vi "Average temperature.vi"() -> ()   [LabVIEW 2019]
panel:
  out "Waveform Chart":cluster{dbl, "Temperature":dbl}(graph)
  in  "Вкл":bool
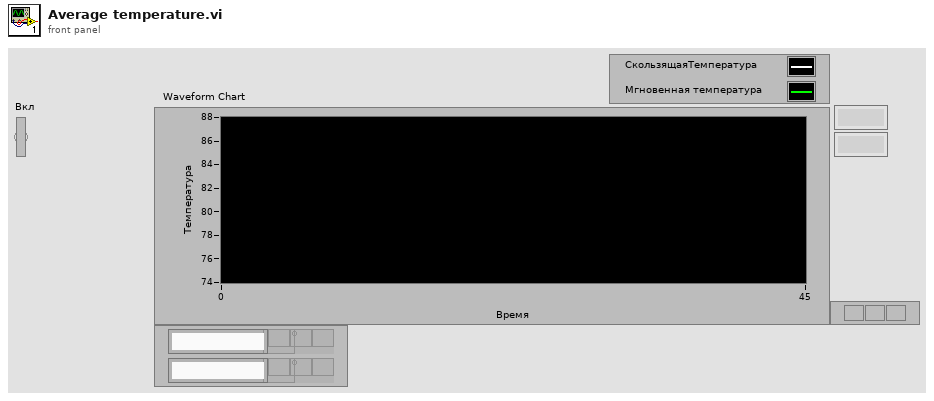
[diagram p1: front panel]
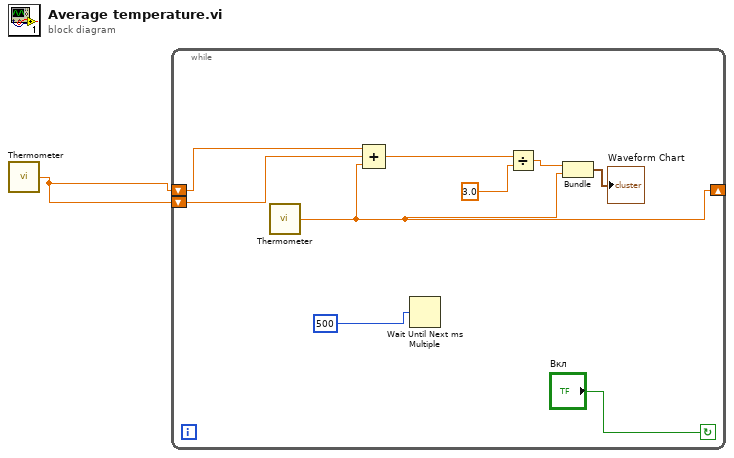
[diagram p0: block diagram]
diagram:
  n1 = call "Thermometer.vi"() -> ("Temperature"=w1:dbl)  [unwired: 1 in]
  n2 = while {
    shift-right: [w3] -> _
    shift-left: w1 -> [w7]
    shift-left: w1 -> [w8]
    stop <- "Вкл" continue-if-true
    n3 = call "Thermometer.vi"() -> ("Temperature"=w3:dbl)  [unwired: 1 in]
    n4 = Compound Arithmetic op=ADD(w7, w8, w3) -> (w6:dbl)
    n5 = Wait Until Next ms Multiple(millisecond multiple=500) -> ()  [unwired: 1 out]
    n6 = Divide(x=w6, y=3.0) -> (x/y=w4:dbl)
    n7 = Bundle(w4, "Temperature"=w3) -> (→"Waveform Chart":cluster{dbl, "Temperature":dbl})  [unwired: 1 in]
  }
